vi "Timer.vi"(6 "Action (Time Elapsed)":T1=enum."TimeElapsed", 8 "error in (no error)":errorcluster, 11 "Time To Elapse":dbl) -> (0 "error out":errorcluster, 1 "Time Elapsed?":bool, 3 "Time Elapsed (s)":dbl)   [LabVIEW 2022 SP3]
doc: "This VI checks whether the Elapsed Time has Elapsed"
uses:
  #typedef_TimerAction.ctl
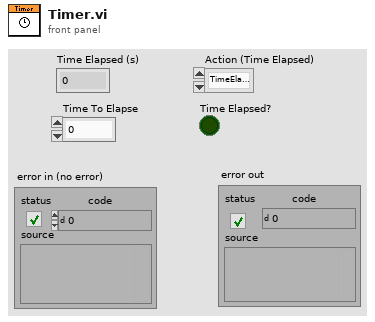
[diagram p1: front panel]
types:
  T1 = typedef "#typedef_TimerAction.ctl" = enum16{"Reset", "TimeElapsed"}
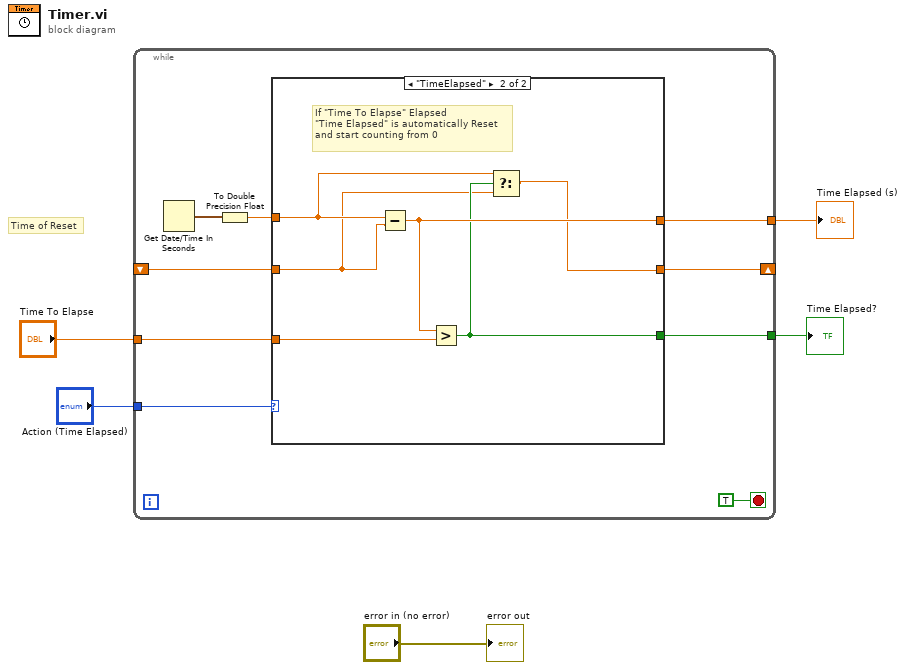
[diagram p0: block diagram]
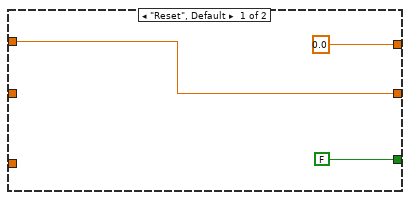
[diagram p2: hidden frame]
diagram:
  # "Time of Reset"
  n1 = while {
    shift-right: [w10] -> _
    shift-left: _ -> [w9]
    tunnel: "Action (Time Elapsed)" -> [w13]
    tunnel: [w8] -> w4
    tunnel: "Time To Elapse" -> [w7]
    tunnel: [w6] -> w1
    stop <- TRUE stop-if-true
    n2 = Get Date/Time In Seconds() -> (seconds since 1Jan1904=w12:timestamp)
    n3 = To Double Precision Float(number=w12) -> (double precision float=w11:dbl)
    n4 = case shown="\"TimeElapsed\"" w13 {
      tunnel: w11 -> [w17 w20]
      tunnel: [w17 w18] -> w10
      tunnel: w9 -> [_ w19]
      tunnel: [0.0 w23] -> w8
      tunnel: w7 -> [_ w22]
      tunnel: [FALSE w21] -> w6
      frame "Reset", Default {
      }
      frame "TimeElapsed" {
        # "If \"Time To Elapse\" Elapsed\n\"Time Elapsed\" is automatically Reset\nand start counting from 0"
        n5 = Subtract(x=w20, y=w19) -> (x-y=w23:dbl)
        n6 = Greater?(x=w23, y=w22) -> (0:w21:bool)
        n7 = Select(t=w20, s=w21, f=w19) -> (s? t:f=w18:dbl)
      }
    }
  }
  "Time Elapsed (s)" <- w4
  "Time Elapsed?" <- w1
  "error out" <- "error in (no error)"
